vi "Make Trap3 position array.vi"(5 "MCL offset scanning range (V)":T1) -> (0 "Scan increment":u64, 1 "Min Y":u64, 2 "Min X":u64, 3 "X Data points":u64, 4 "Y data points":u64)   [LabVIEW 2014]
panel:
  out "Array":dbl[][](array[numeric])
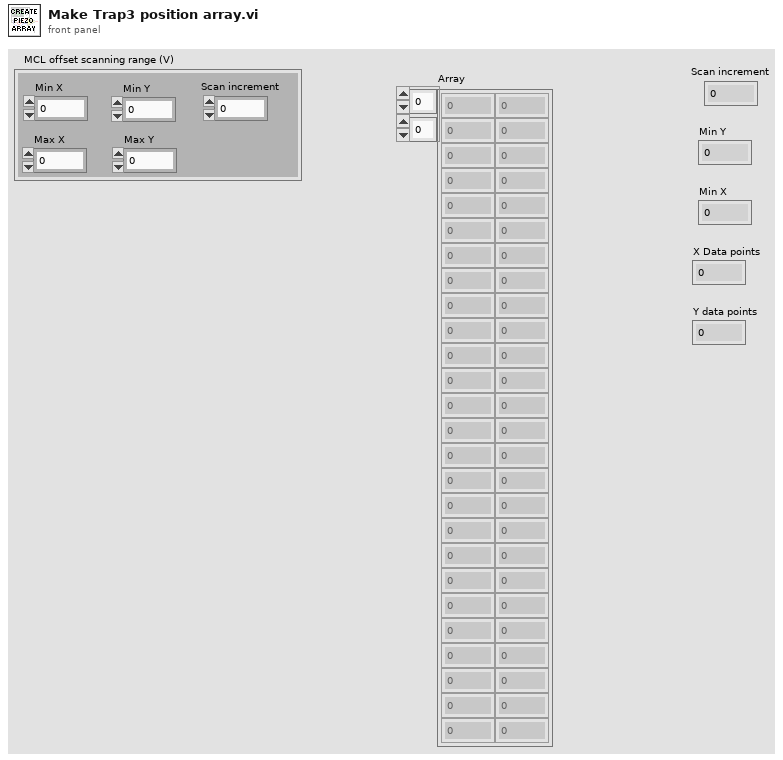
[diagram p1: front panel]
types:
  T1 = cluster{"Min X":dbl, "Max X":dbl, "Min Y":dbl, "Max Y":dbl, "Scan increment":dbl}
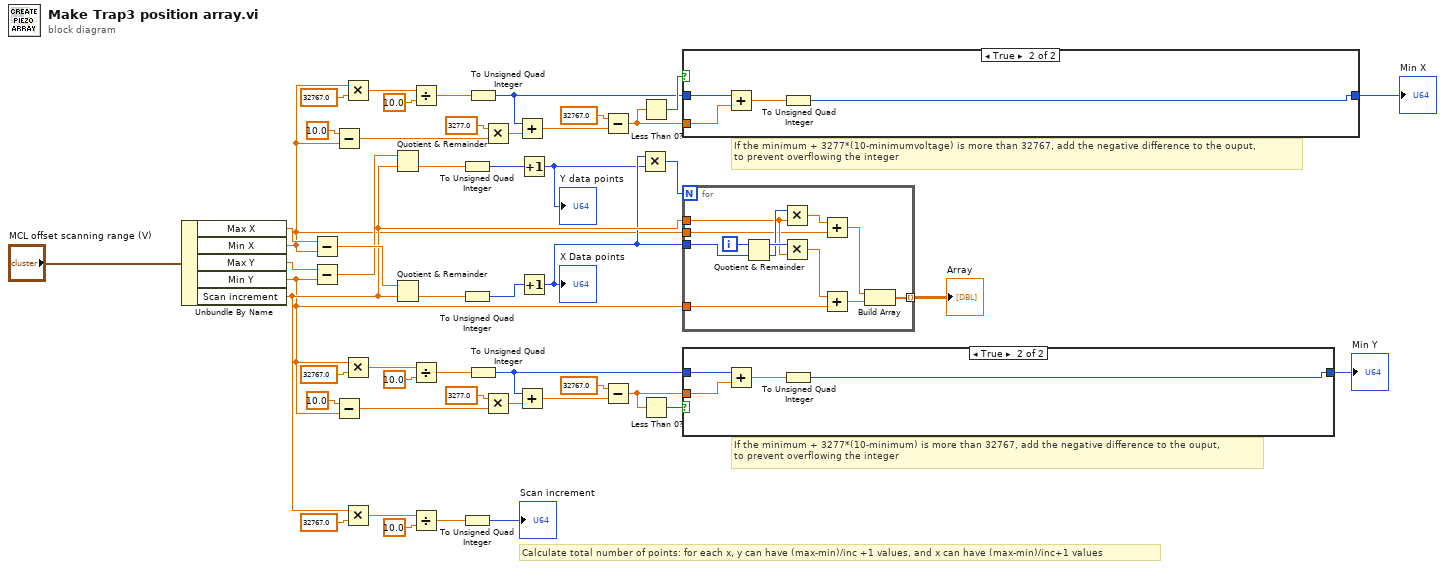
[diagram p0: block diagram]
diagram:
  # "If the minimum + 3277*(10-minimum) is more than 32767, add the negative difference to the ouput,\nto prevent overflowing the integer"
  # "If the minimum + 3277*(10-minimumvoltage) is more than 32767, add the negative difference to the ouput,\nto prevent overflowing the integer"
  # "Calculate total number of points: for each x, y can have (max-min)/inc +1 values, and x can have (max-min)/inc+1 values"
  n1 = Unbundle By Name("MCL offset scanning range (V)") -> ("Max X"=w48:dbl, "Min X"=w1:dbl, "Max Y"=w45:dbl, "Min Y"=w2:dbl, "Scan increment"=w31:dbl)
  n2 = Subtract(x=w48, y=w1) -> (x-y=w47:dbl)
  n3 = Subtract(x=w45, y=w2) -> (x-y=w44:dbl)
  n4 = Subtract(x=10.0 ("y"), y=w1) -> (x-y=w20:dbl)
  n5 = Subtract(x=10.0 ("y"), y=w2) -> (x-y=w12:dbl)
  n6 = Multiply(x=w1, y=32767.0) -> (x*y=w34:dbl)
  n7 = Multiply(x=w2, y=32767.0) -> (x*y=w27:dbl)
  n8 = Multiply(x=w31, y=32767.0) -> (x*y=w37:dbl)
  n9 = Quotient & Remainder(x=w44, y=w31) -> (floor(x/y)=w43:dbl)  [unwired: 1 out]
  n10 = Quotient & Remainder(x=w47, y=w31) -> (floor(x/y)=w41:dbl)  [unwired: 1 out]
  n11 = Divide(x=w34, y=10.0) -> (x/y=w33:dbl)
  n12 = Divide(x=w27, y=10.0) -> (x/y=w28:dbl)
  n13 = Divide(x=w37, y=10.0) -> (x/y=w38:dbl)
  n14 = To Unsigned Quad Integer(1:w43) -> (0:w42:u64)
  n15 = To Unsigned Quad Integer(1:w41) -> (0:w46:u64)
  n16 = To Unsigned Quad Integer(1:w38) -> (0:→"Scan increment":u64)
  n17 = To Unsigned Quad Integer(1:w33) -> (0:w8:u64)
  n18 = To Unsigned Quad Integer(1:w28) -> (0:w3:u64)
  n19 = Multiply(x=3277.0, y=w20) -> (x*y=w7:dbl)
  n20 = Multiply(x=3277.0, y=w12) -> (x*y=w5:dbl)
  n21 = Add(x=w8, y=w7) -> (x+y=w6:dbl)
  n22 = Add(x=w3, y=w5) -> (x+y=w4:dbl)
  n23 = Increment(x=w42) -> (x+1=w23:u64)
  "Y data points" <- w23
  n24 = Increment(x=w46) -> (x+1=w24:u64)
  "X Data points" <- w24
  n25 = Subtract(x=32767.0 ("y"), y=w6) -> (x-y=w17:dbl)
  n26 = Subtract(x=32767.0 ("y"), y=w4) -> (x-y=w15:dbl)
  n27 = Multiply(x=w24, y=w23) -> (x*y=w25:u64)
  n28 = Less Than 0?(x=w17) -> (x < 0?=w18:bool)
  n29 = Less Than 0?(x=w15) -> (x < 0?=w14:bool)
  n30 = case shown="True" w18 {
    tunnel: w17 -> [_ w53]
    tunnel: w8 -> [w50 w54]
    tunnel: [w50 w51] -> w16
    frame False {
    }
    frame True {
      n31 = Add(x=w54, y=w53) -> (x+y=w52:dbl)
      n32 = To Unsigned Quad Integer(1:w52) -> (0:w51:u64)
    }
  }
  "Min X" <- w16
  n33 = for {
    N: w25 -> [_]
    tunnel: w24 -> [w65]
    tunnel: w31 -> [w62]
    tunnel: w1 -> [w59]
    tunnel: w2 -> [w58]
    tunnel: [w55] -> w40 mode=indexing
    i -> [w66]
    n34 = Quotient & Remainder(x=w66, y=w65) -> (x-y*floor(x/y)=w64:u64, floor(x/y)=w63:u64)
    n35 = Multiply(x=w63, y=w62) -> (x*y=w60:dbl)
    n36 = Multiply(x=w64, y=w62) -> (x*y=w61:dbl)
    n37 = Add(x=w60, y=w59) -> (x+y=w57:dbl)
    n38 = Add(x=w61, y=w58) -> (x+y=w56:dbl)
    n39 = Build Array(w57, w56) -> (w55:dbl[])
  }
  "Array" <- w40
  n40 = case shown="True" w14 {
    tunnel: w15 -> [_ w70]
    tunnel: w3 -> [w67 w71]
    tunnel: [w67 w68] -> w9
    frame False {
    }
    frame True {
      n41 = Add(x=w71, y=w70) -> (x+y=w69:dbl)
      n42 = To Unsigned Quad Integer(1:w69) -> (0:w68:u64)
    }
  }
  "Min Y" <- w9
